vi "Set Single-Line Package Attribute Value.vi"(6 "add nonexisting attribute to string (T)":bool=TRUE, 8 "error in (no error)":errorcluster, 9 "package attribute value":string, 10 "package attribute name":string, 11 "package attributes string in":string) -> (0 "error out":errorcluster, 1 "attribute found?":bool, 2 "new attribute added to string?":bool, 3 "package attributes string out":string)   [LabVIEW 2014, in "NIPM_API.lvlib"]
doc: "Sets the value for an attribute in a package attribute string.\n\npackage attributes string in - This is the initial string containing the package attributes. For example, this string could come from reading the contents of an unpacked package's control file.\n\npackage attribute name - This is the name of the attribute whose value you want to change.\n\npackage attribute value - This is the value you want to set the attribute to.\n\nadd nonexisting attribute to string - If this VI does not find the \"package attribute name\" in the \"package attributes string in\" string, this input determines whether this VI will add the \"package attribute name\" and \"package attribute value\" to the \"package attribute string\".\nNote: If this input is TRUE, but the \"package attribute value\" is a default value (\"\"), then this VI will not add a new attribute to the string.\n\nnew attribute added to string? - This output will be TRUE if a new attribute (did not exist in the incoming \"package attributes string in\" string) was added to the package attributes string.\n\nattribute found? - This output will be TRUE if the \"package attribute name\" was found in the incoming \"package attributes string in\" string."
uses:
  NIPM_API.lvlib
  <vilib>/Utility/error.llb/whitespace.ctl
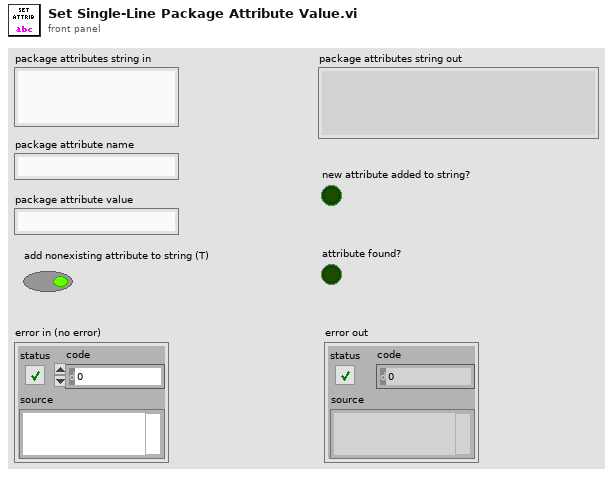
[diagram p1: front panel]
types:
  T1 = typedef "whitespace.ctl" = u16
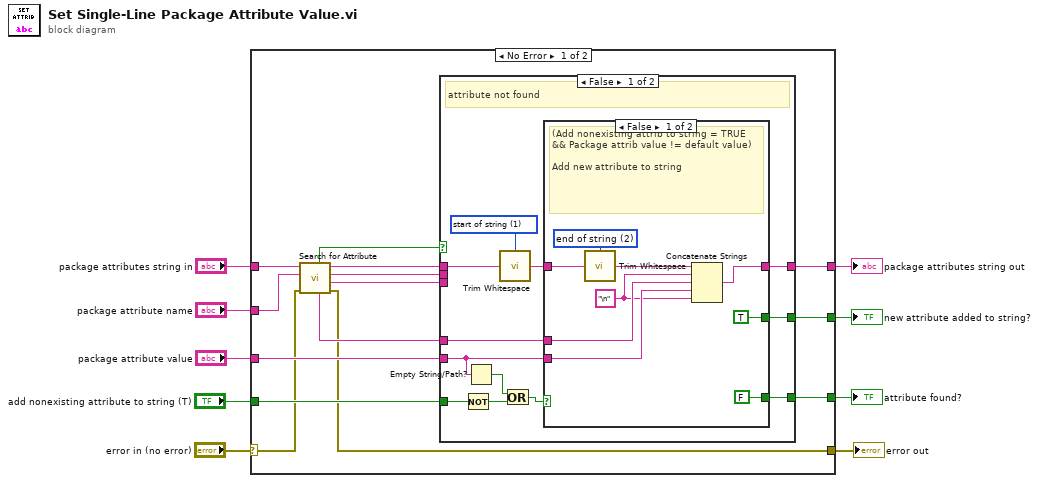
[diagram p0: block diagram]
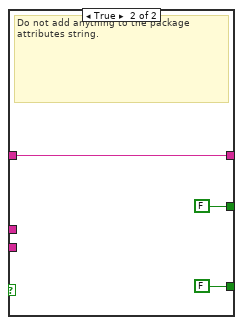
[diagram p2: hidden frame]
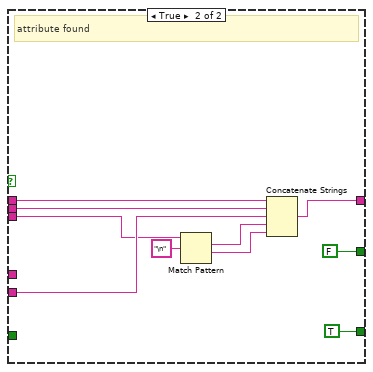
[diagram p3: hidden frame]
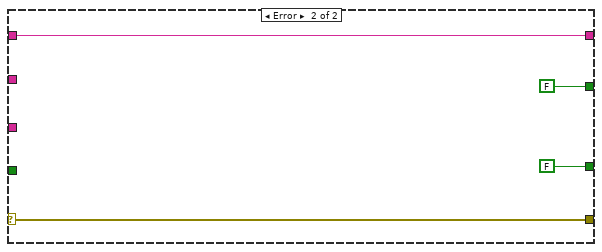
[diagram p4: hidden frame]
diagram:
  n1 = case shown="No Error" "error in (no error)" {
    selector: "error in (no error)" -> [w11 w61]
    tunnel: [w22 w58] -> w9
    tunnel: "package attribute name" -> [w17 _]
    tunnel: "package attributes string in" -> [w18 w58]
    tunnel: [w10 w61] -> w5
    tunnel: "package attribute value" -> [w23 _]
    tunnel: [w21 FALSE] -> w3
    tunnel: "add nonexisting attribute to string (T)" -> [w20 _]
    tunnel: [w19 FALSE] -> w1
    frame No Error {
      n2 = call "Search for Attribute.vi"("error in (no error)"=w11, "package attribute name"=w17, "package attributes CLI string in"=w18) -> ("error out"=w10:errorcluster, "string after attribute"=w14:string, "string matching attribute"=w15:string, "string before attribute"=w16:string, "package attribute string"=w12:string, "attribute found?"=w13:bool)  [unwired: 3 in]
      n3 = case shown="False" w13 {
        tunnel: w16 -> [w35 w57]
        tunnel: w15 -> [_ w56]
        tunnel: w23 -> [w27 w55]
        tunnel: w14 -> [_ w54]
        tunnel: [w33 w52] -> w22
        tunnel: [w34 FALSE] -> w21
        tunnel: w12 -> [w32 _]
        tunnel: w20 -> [w28 _]
        tunnel: [w31 TRUE] -> w19
        frame False {
          w24 = T1 1 items=["both", "start of string", "end of string"] ("location (both)")
          # "attribute not found"
          n4 = Not(x=w28) -> (.not. x?=w30:bool)
          n5 = Empty String/Path?(string/path=w27) -> (empty?=w29:bool)
          n6 = call <vilib>:"Trim Whitespace.vi"("string"=w35, "location (both)"=w24) -> ("trimmed string"=w25:string)
          n7 = Or(x=w29, y=w30) -> (x .or. y?=w26:bool)
          n8 = case shown="False" w26 {
            tunnel: w25 -> [w44 w47]
            tunnel: [TRUE FALSE] -> w34
            tunnel: [w42 w47] -> w33
            tunnel: w32 -> [w41 _]
            tunnel: w27 -> [w40 _]
            tunnel: [FALSE FALSE] -> w31
            frame False {
              w37 = "\n"
              w38 = T1 2 items=["both", "start of string", "end of string"] ("location (both)")
              # "(Add nonexisting attrib to string = TRUE && Package attrib value != default value)\n\nAdd new attribute to string"
              n9 = call <vilib>:"Trim Whitespace.vi"("string"=w44, "location (both)"=w38) -> ("trimmed string"=w39:string)
              n10 = Concatenate Strings(w39, w37, w41, w40, w37) -> (w42:string)
            }
            frame True {
              # "Do not add anything to the package attributes string."
            }
          }
        }
        frame True {
          # "attribute found"
          n11 = Match Pattern(string=w54, regular expression="\n") -> (match substring=w50:string, after substring=w49:string)  [unwired: 1 in, 2 out]
          n12 = Concatenate Strings(w57, w56, w55, w50, w49) -> (w52:string)
        }
      }
    }
    frame Error {
    }
  }
  "package attributes string out" <- w9
  "error out" <- w5
  "new attribute added to string?" <- w3
  "attribute found?" <- w1
